vi "YAV Z485噪音分贝采集.vi"(0 "VISA resource name":refnum<visa-resource-name>="COM1" caption="端口") -> ()   [LabVIEW 2014]
doc: "高级串行读取和写入范例可执行串口读取、串口写入或者串口读写操作，同时可设置串口高级功能，例如缓冲区大小、终止符和XON/XOFF流控制等。用户可在前面板选择操作（读取或写入）。如果选择全部，VI将写入数据并读取数据，然后关闭开放给端口的VISA会话句柄。\n\n串口的参数组必须匹配连接仪器或设备的参数。在本范例中，待读取字节参数可指定串口读取的字节数。如端口字节超过指定的字节数，超出部分将不会被读取。如果指定读取的字节数超过实际字节数，可能返回超时错误。\n\n步骤：\n1) 选择串行资源并配置参数（波特率、数据位、奇偶、停止位和流控制）。\n2) 可以启用并设置终止符。运行本范例前先设置所需输入缓冲区大小。\n3) 选择需执行的操作。\n4) 连接串口至设备。如未发现可用设备，请按以下任一方式执行环回测试。在RS-232线缆中短路引脚2和3，或者在RS-485/422线缆中短路引脚4和8以及引脚5和9。\n5) 运行VI并查看读取的数据。（如果已执行环回测试，“读取字符串”将匹配“写入字符串”。）\n\n本范例说明的部分高级功能可能有利于用户的应用程序开发。应用程序并不需要使用范例中的全部功能。设置输入缓冲区大小对应用程序十分重要。本范例可扩展流控制选项以包括XON和XOFF，从而允许用户选择控制字符。在前面板中显示超时参数，以便于用户指定VISA读取等待指定字节数的超时时间。同时用户可使用多种方式控制结束符，请查看后续说明。\n\n请注意在运行范例时，用户可以单击写入或读取按钮并更改读取字节参数的值。但对于其它参数，必须先停止该范例才能进行修改。\n\n将I/O缓冲区大小设置为超出预期接收数据总数。这将有利于不使用流控制的应用程序，因为当接收缓冲区溢出时可能会丢失字符。\n\n设置超时时间，确保当操作在指定时间内无法完成时可返回一个超时错误。\n\n部分设备需要通过终止符确定命令字符串的结束位置。部分设备将发送终止符以说明待读取数据的末端。\n\n本范例将说明当缓冲区中发现结束符时如何结束读取操作或者添加结束符至写入数据的末端。如需启用读取至终止符，可使用“VISA配置串口”函数或者用于读取、结束符启用和结束符的VISA属性串口结束模式。如需使用终止符结束写入，可使用写入、发送结束启用和结束符的VISA属性串口结束模式。在本范例中，读取和写入操作将使用相同的终止符。在应用程序中也可以指定两个不同的终止符。\n\n用户的应用程序可能需要特定字符用于XON/XOFF流控制。通过VISA属性流控制XOFF字符和流控制XON字符可以指定该字符。请注意如使用标准XON和XOFF字符，无法将十进制17和19作为数据值。同时使用流控制并设置正确的缓冲区大小可避免缓冲区溢出。"
uses:
  <vilib>/Instr/_visa.llb/VISA Configure Serial Port (Instr).vi
panel:
  in  "选项卡控件":enum32{"显示", "说明"}(tab)
  out "分贝值":dbl format="%.1f"
  in  "波特率":u32=9600
  out "波形图表":dbl(graph)
  in  "发送":string="\u0001\u0003\u0000\u0001\u0000\u0001帐"
  out "接收":string
  in  "stop":bool caption="停止"
  # "YAV Z485噪音分贝采集"
  # "亚为科技 www.yav123.com"
  # "一定要安装NIVISA，百度一下。串口号只可选择，不可强行输入，选择不了证明没安装NIVISA"
  # "1、本程序兼容modbus rtu指令和YAV字符串指令\n2、噪音数据01寄存器，可03指令读取\n3、ID在02寄存器，波特率在03寄存器，可用modbus调试助手，06指令设置\n4、波特率默认为9600，例如设置115200，在03寄存器写入1152的十六进制即可。01 06 00 03 04 80 7A AA\n5、不管哪种协议，上电会自动发送一段字符串，显示屏的ID。如果ASC模式下显示为乱码，则波特率设置不正确，更换其他\n波特率测试即可。"
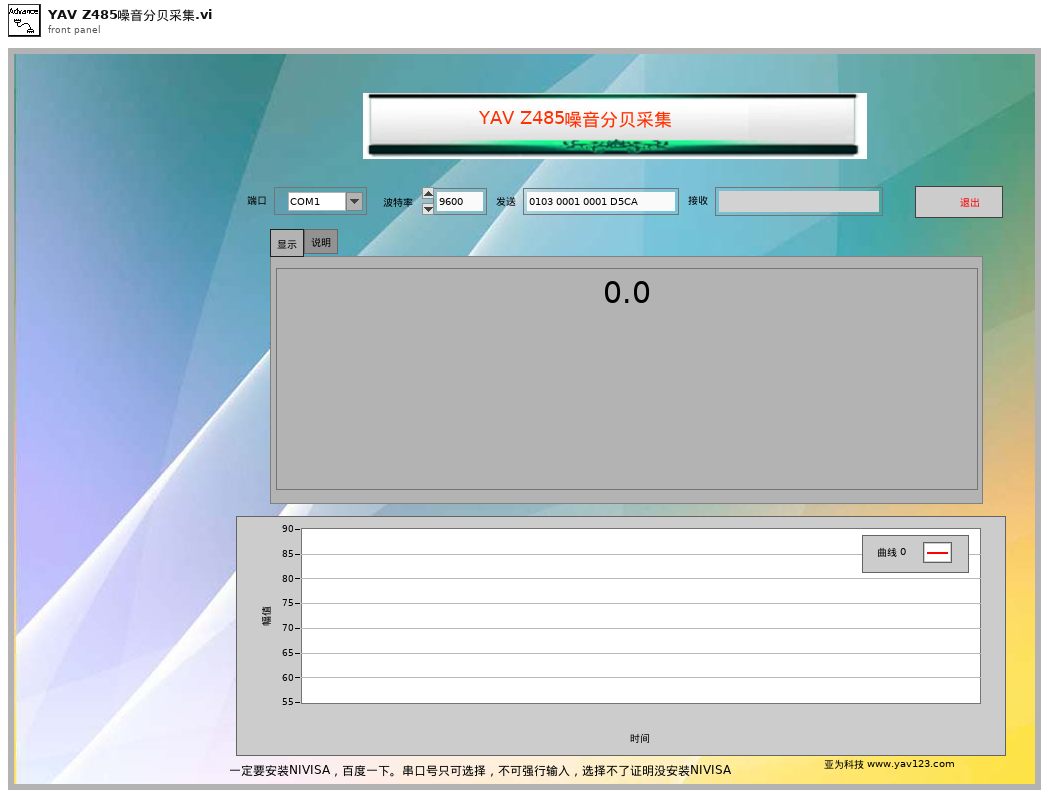
[diagram p1: front panel]
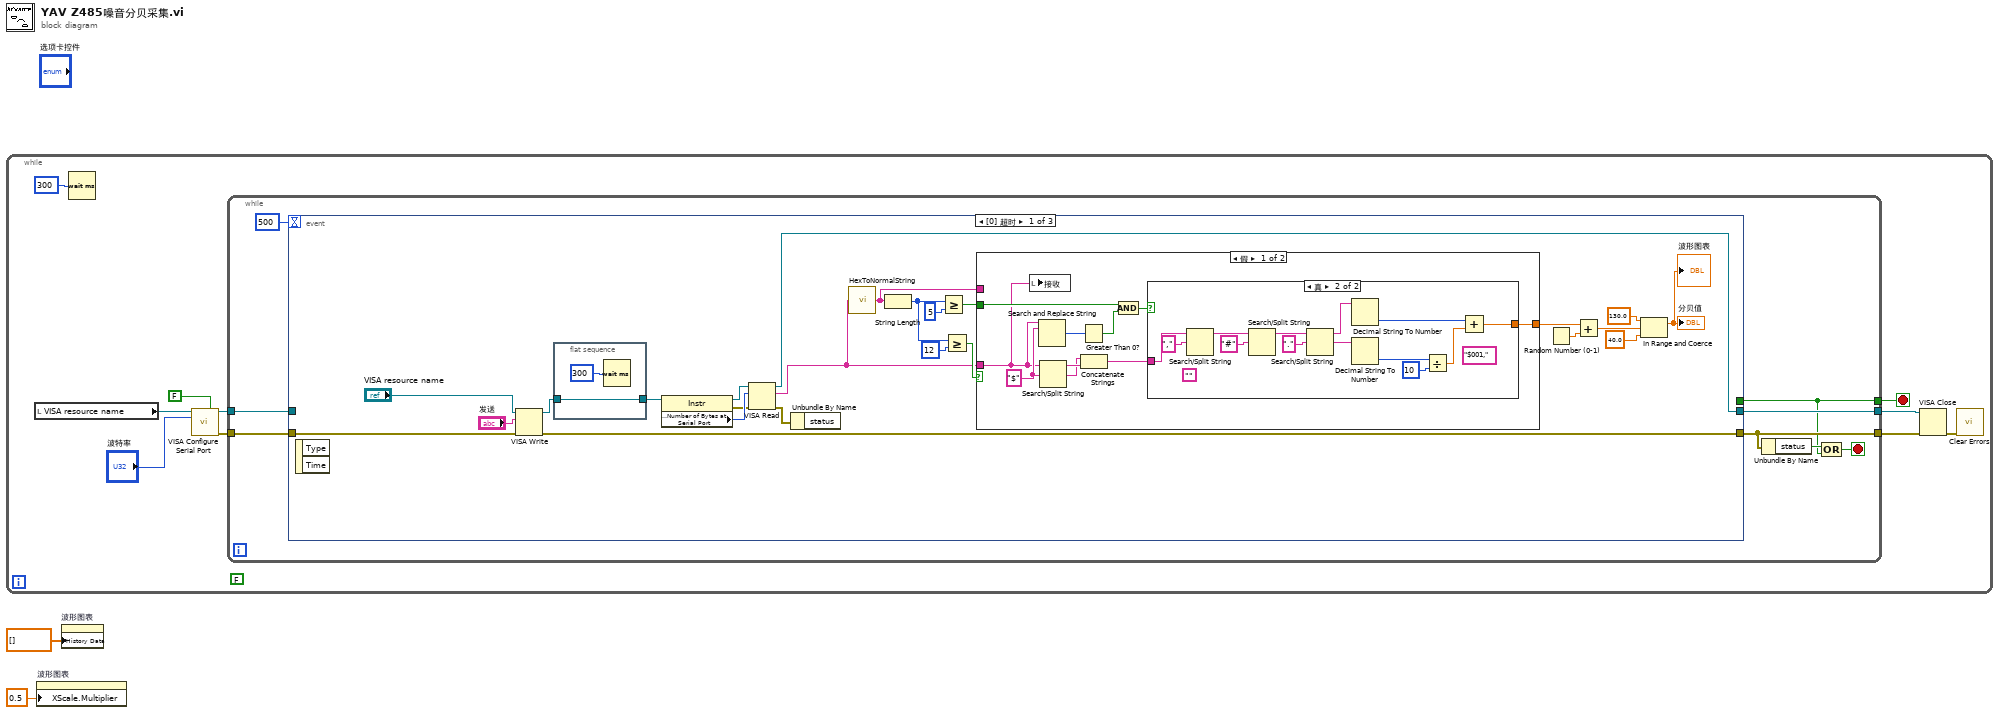
[diagram p0: block diagram]
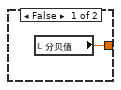
[diagram p2: hidden frame]
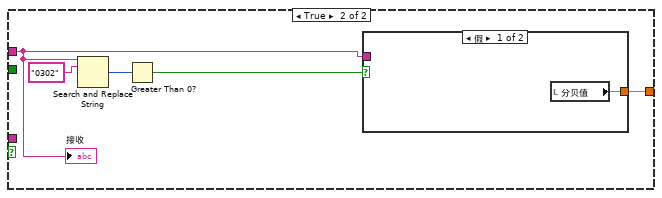
[diagram p3: hidden frame]
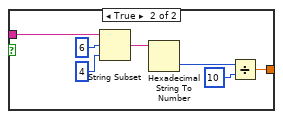
[diagram p4: hidden frame]
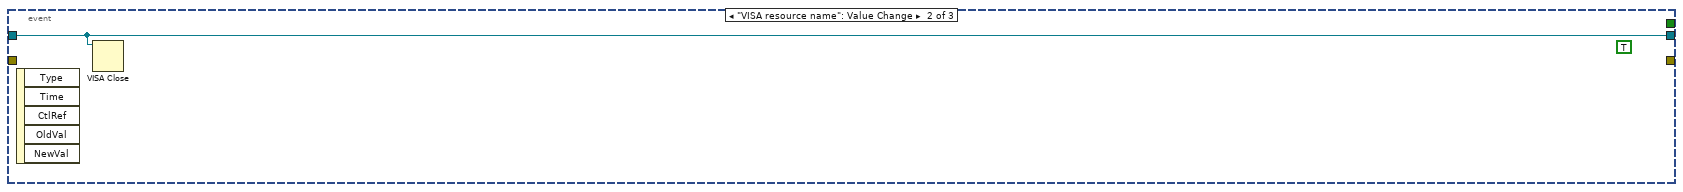
[diagram p5: hidden frame]
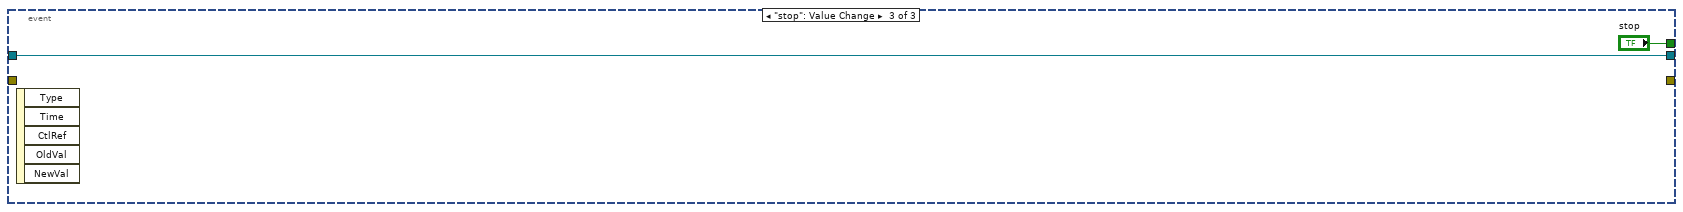
[diagram p6: hidden frame]
diagram:
  n1 = while {
    stop <- w9 stop-if-true
    (unwired) FALSE
    n2 = local read "VISA resource name"() -> (w4:refnum<visa-resource-name>)
    n3 = Wait (ms)(milliseconds to wait=u32 300 ("等待时间（毫秒）")) -> ()  [unwired: 1 out]
    n4 = call-poly "VISA Configure Serial Port"("VISA resource name"=w4, "Enable Termination\nChar (T)"=FALSE ("Enable Termination\nChar (T)"), "baud rate (9600)"="波特率") -> ("VISA resource name out"=w6:refnum<visa-resource-name>, "error out"=w5:errorcluster)  [unwired: 7 in, 4 out]
    n5 = while {
      tunnel: w6 -> [w19]
      tunnel: [w17] -> w12
      tunnel: [w13] -> w9
      tunnel: w5 -> [w18]
      tunnel: [w16] -> w11
      stop <- w15 stop-if-true
      n6 = event shown="[0] 超时" {
        selector: _ -> [_ _ _]
        dyn-events: _ -> [_ _ _]
        timeout: 500 -> [_ _ _]
        tunnel: w19 -> [_ w84 w85]
        tunnel: w18 -> [w43 _ _]
        tunnel: [w42 w84 w85] -> w17
        tunnel: [w32 _ _] -> w16
        tunnel: [_ _ "stop"] -> w13
        event Timeout {
          n7 = event-data() -> ()  [unwired: 1 in, 2 out]
          n8 = VISA Write(VISA resource name="VISA resource name", write buffer="发送", error in (no error)=w43) -> (VISA resource name out=w44:refnum<visa-resource-name>, error out=w32:errorcluster)  [unwired: 1 out]
          n9 = flat-sequence {
            tunnel: w44 -> [w82]
            tunnel: [w82] -> w28
            frame #0 {
              n10 = Wait (ms)(milliseconds to wait=u32 300 ("等待时间（毫秒）")) -> ()  [unwired: 1 out]
            }
          }
          n11 = property class="Instr"(reference=w28) -> (reference out=w27:refnum<visa-resource-name>, error out=w26:errorcluster, "Serial Settings:Number of Bytes at Serial Port"=w37:u32)  [unwired: 1 in]
          n12 = VISA Read(VISA resource name=w27, byte count=w37, error in (no error)=w26) -> (VISA resource name out=w42:refnum<visa-resource-name>, read buffer=w36:string, error out=w38:errorcluster)  [unwired: 1 out]
          n13 = Unbundle By Name(w38) -> ()  [unwired: 1 out]
          n14 = call "HexToNormalString.vi"("Hex Display"=w36) -> ("Normal Display"=w21:string)  [unwired: 14 in]
          n15 = String Length(string=w21) -> (length=w30:i32)
          n16 = Greater Or Equal?(x=w30, y=5) -> (x >= y?=w29:bool)
          n17 = Greater Or Equal?(x=w30, y=12) -> (x >= y?=w39:bool)
          n18 = case shown="假" w39 {
            tunnel: w36 -> [w45 _]
            tunnel: [w54 w73] -> w23
            tunnel: w29 -> [w51 _]
            tunnel: w21 -> [_ w69]
            frame False {
              w49 = "$"
              n19 = local write "接收"(w45) -> ()
              n20 = Search and Replace String(input string=w45, search string=w49) -> (number of replacements=w53:i32)  [unwired: 6 in, 3 out]
              n21 = Search/Split String(string=w45, search string/char (-)=w49) -> (substring before match=w48:string, match + rest of string=w47:string)  [unwired: 1 in, 1 out]
              n22 = Greater Than 0?(x=w53) -> (x > 0?=w52:bool)
              n23 = Concatenate Strings(w47, w48) -> (w46:string)
              n24 = And(x=w51, y=w52) -> (x .and. y?=w50:bool)
              n25 = case shown="真" w50 {
                tunnel: w46 -> [_ w68]
                tunnel: [w55 w56] -> w54
                frame False {
                  n26 = local read "分贝值"() -> (w55:dbl)
                }
                frame True {
                  (unwired) "$001,"
                  (unwired) ""
                  n27 = Search/Split String(string=w68, search string/char (-)=",") -> (substring before match=w59:string)  [unwired: 1 in, 2 out]
                  n28 = Search/Split String(string=w59, search string/char (-)="#") -> (substring before match=w57:string)  [unwired: 1 in, 2 out]
                  n29 = Search/Split String(string=w57, search string/char (-)=".") -> (substring before match=w65:string, match + rest of string=w64:string)  [unwired: 1 in, 1 out]
                  n30 = Decimal String To Number(string=w65) -> (number=w61:i32)  [unwired: 2 in, 1 out]
                  n31 = Decimal String To Number(string=w64) -> (number=w63:i32)  [unwired: 2 in, 1 out]
                  n32 = Divide(x=w63, y=10) -> (x/y=w60:dbl)
                  n33 = Add(x=w61, y=w60) -> (x+y=w56:dbl)
                }
              }
            }
            frame True {
              n34 = Search and Replace String(input string=w69, search string="0302" ("搜索字符串")) -> (number of replacements=w71:i32)  [unwired: 6 in, 3 out]
              n35 = Greater Than 0?(x=w71) -> (x > 0?=w70:bool)
              n36 = case shown="假" w70 {
                tunnel: [w74 w76] -> w73
                tunnel: w69 -> [_ w75]
                frame False {
                  n37 = local read "分贝值"() -> (w74:dbl)
                }
                frame True {
                  n38 = String Subset(string=w75, offset (0)=6, length (rest)=4) -> (substring=w80:string)
                  n39 = Hexadecimal String To Number(string=w80) -> (number=w77:u32)  [unwired: 2 in, 1 out]
                  n40 = Divide(x=w77, y=u32 10) -> (x/y=w76:dbl)
                }
              }
              "接收" <- w69
            }
          }
          n41 = Random Number (0-1)() -> (number: 0 to 1=w24:dbl)
          n42 = Add(x=w23, y=w24) -> (x+y=w22:dbl)
          n43 = In Range and Coerce(upper limit=130.0 ("上限"), x=w22, lower limit=40.0 ("下限")) -> (coerced(x)=→"分贝值" →"波形图表":dbl)  [unwired: 1 out]
        }
        event "VISA resource name": Value Change {
          (unwired) TRUE ("stop")
          n44 = event-data() -> ()  [unwired: 1 in, 5 out]
          n45 = VISA Close(VISA resource name=w84) -> ()  [unwired: 1 in, 1 out]
        }
        event "stop": Value Change {
          n46 = event-data() -> ()  [unwired: 1 in, 5 out]
        }
      }
      n47 = Unbundle By Name(w16) -> ("status"=w20:bool)
      n48 = Compound Arithmetic op=OR(w20, w13) -> (w15:bool)
    }
    n49 = VISA Close(VISA resource name=w12, error in (no error)=w11) -> (error out=w10:errorcluster)
    n50 = call <vilib>:"Clear Errors.vi"("error in (no error)"=w10) -> ()  [unwired: 5 in, 2 out]
  }
  n51 = property on="波形图表" class="WFChart (严格)"("XScale.Multiplier"=0.5 ("X标尺.偏移量与缩放系数:缩放系数")) -> ()  [unwired: 2 in, 2 out]
  n52 = property on="波形图表" class="WFChart (严格)"("History Data"=dbl[] [] ("历史数据")) -> ()  [unwired: 2 in, 2 out]
